vi "DMCConfiguatorGui.vi"() -> ()   [LabVIEW 2016]
uses:
  DMCConfiguatorGui.TypeGui.ctl
  DMCConfiguatorGui.VarGui.ctl
  DMCConfiguatorGui.ConfigData.ctl
  DMCConfiguatorGui.Component.ctl
  DMCConfiguatorGui.Type.ctl
  DMCConfiguatorGui.Var.ctl
  Logger/Logger.Variant.Sets.ctl
  Station/Station.Changeover.State.vi
  Station/Station.Plate.Properties.ctl
  Sequence/Sequence.Code.SerialFormat.ctl
  Drivers/V7310/LowLevel/V7310.Job.Sets.ctl
  Sequence/Sequence.PlateType.ctl
  DMCConfiguatorGui.Action.ctl
  <vilib>/Utility/miscctls.llb/LVRowAndColumnUnsignedTypeDef.ctl
  <vilib>/Utility/miscctls.llb/LVRowAndColumnTypeDef.ctl
  tools/Translator/Translator.Message.ctl
  tools/CitTemplate/citTemplate.errData.ctl
  tools/EventLog/EventLog.EventSource.ctl
  tools/Config/Config.Global.vi
  Global/ApplicationGlobal.vi
  Station/Station.Global.vi
panel:
  out "DMCconfig":i32
  out "Plate":T1
  in  "Components":i32(listbox) caption="Komponenty"
  in  "ConfigAdd":bool
  in  "ConfigInUse":i32(ring) caption="Konfiguracja" items=["Default", "975 009 005 0", "APU", "4801020307", "4801020607", "480102040R", "ceTCV", "M.KÊSKA", "cTCV", "probny", "ctcv_nrzaworu", "scania"]
  out "OrderSets":T2={"State"=enum."Init", "ImgPath"=path "", "WabcoPlate"="", "WabcoProduct"="", "ClientProduct"="", "ClientPlate"="", "TotalQuantity"=0, "OrderQuantity"=0, "Serial"=0, "Wabco"={"LaserJob"="", "AdditionalTxt"="", "FactoryCode"="037", "RevID"=0, "ForkID"=0, "FailuresLimit"=0, "GlobalCnt"=0, "ScannerProgram"=0, "SerialFormat"=enum."6 dig", "CoordA"={"X"=0.0, "Y"=0.0, "Angle"=0.0}, "CoordB"={"X"=0.0, "Y"=0.0, "Angle"=0.0}, "DMCconfig"=0, "CVX_Program"=0}, "Client"={"LaserJob"="", "AdditionalTxt"="", "FactoryCode"="037", "RevID"=0, "ForkID"=0, "FailuresLimit"=0, "GlobalCnt"=0, "ScannerProgram"=0, "SerialFormat"=enum."6 dig", "CoordA"={"X"=0.0, "Y"=0.0, "Angle"=0.0}, "CoordB"={"X"=0.0, "Y"=0.0, "Angle"=0.0}, "DMCconfig"=0, "CVX_Program"=0}}
  out "ConfigData":T7[](array[typedef])
  in  "Hider":bool
  in  "ClearAll":bool
  out "CreateDate":string
  in  "Cancel":bool
  in  "Save":bool
  in  "Down":bool
  in  "Up":bool
  in  "ConfigName":string caption="Nazwa"
  in  "ConfigDelete":bool
  out "_loop":i32(ring)=4
  in  "Delete":bool
  in  "Add":bool
  in  "Variable":T11
  in  "Text":string
  in  "Type":T12 caption="Typ"
  out "DMC":string caption="DMC (#32)"
  out "Panel":refnum<vi>
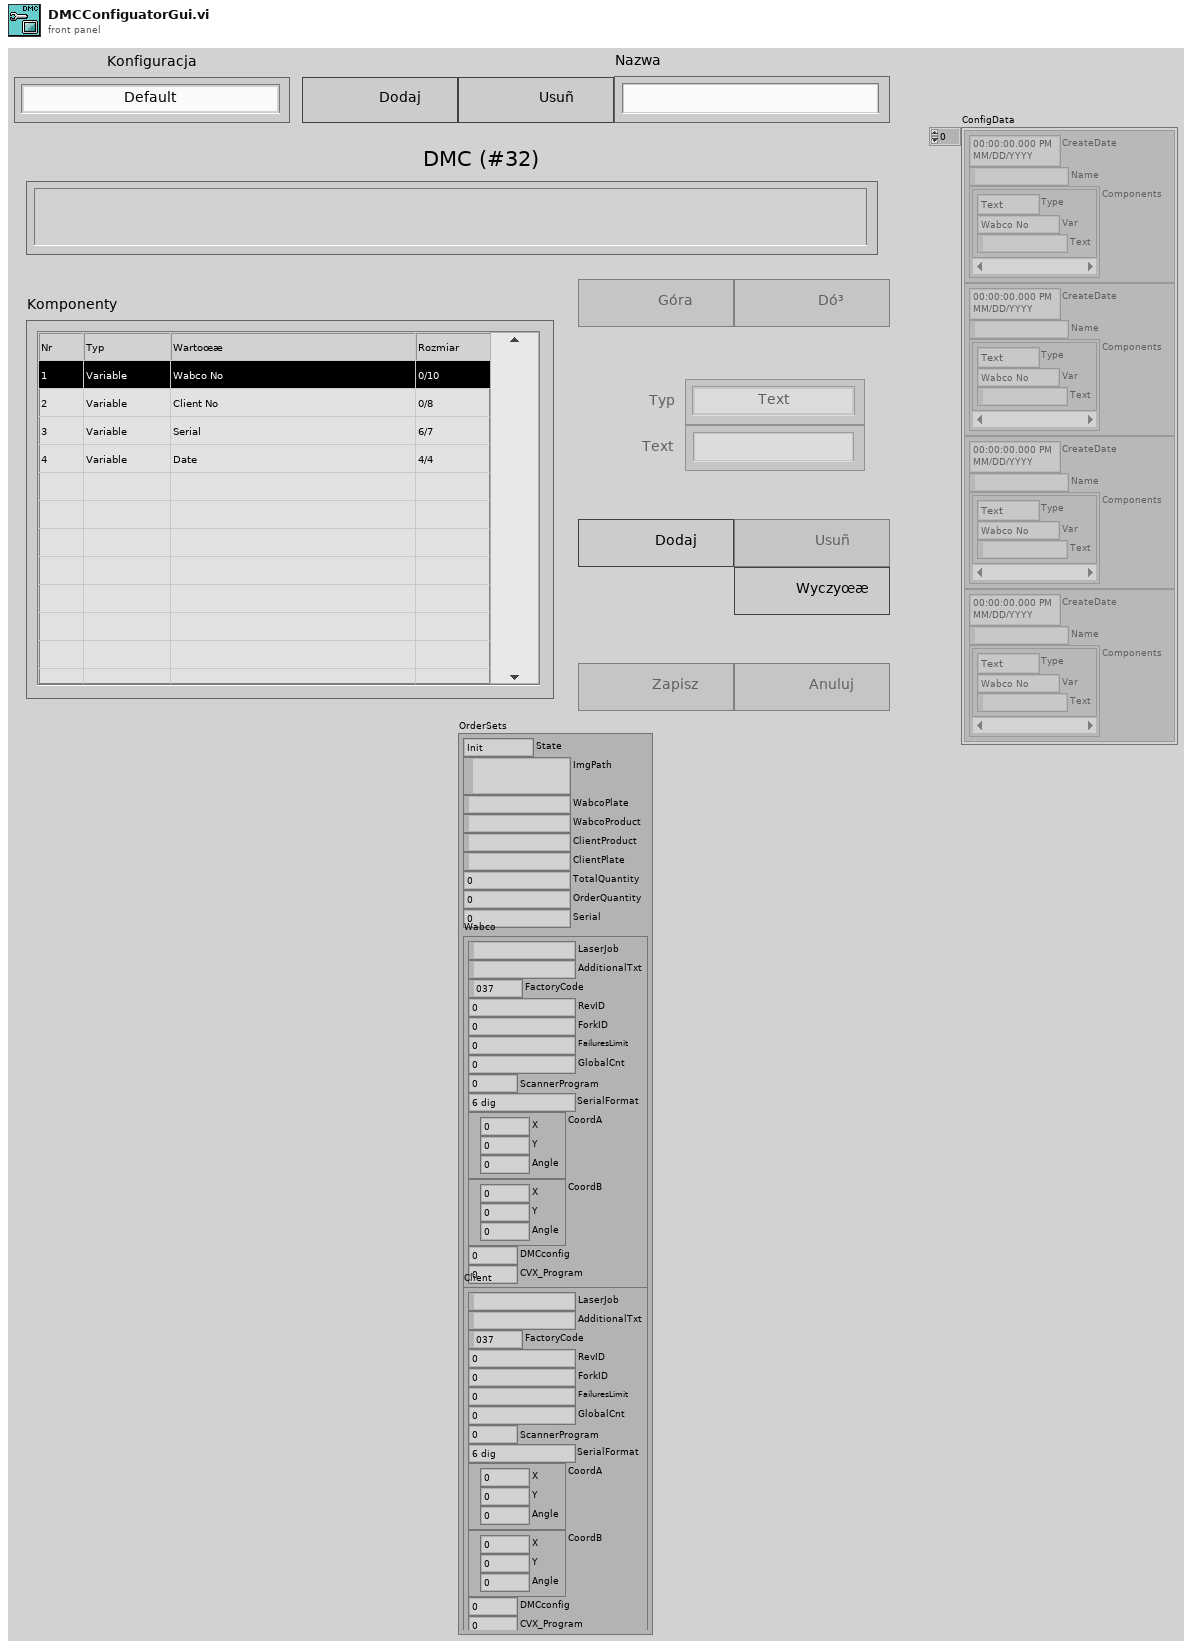
[diagram p1: front panel]
types:
  T1 = typedef "Sequence.PlateType.ctl" = enum16{"Wabco", "Client"}
  T2 = typedef "Logger.Variant.Sets.ctl" = cluster{"State":T3, "ImgPath":path, "WabcoPlate":string, "WabcoProduct":string, "ClientProduct":string, "ClientPlate":string, "TotalQuantity":u16, "OrderQuantity":u16, "Serial":i32, "Wabco":T4, "Client":T4}
  T3 = typedef "Station.Changeover.State.vi" = enum16{"Init", "Scaning", "NOK", "Wait for ack", "Ready"}
  T4 = typedef "Station.Plate.Properties.ctl" = cluster{"LaserJob":string, "AdditionalTxt":string, "FactoryCode":string, "RevID":u8, "ForkID":u8, "FailuresLimit":u16, "GlobalCnt":i32, "ScannerProgram":u8, "SerialFormat":T5, "CoordA":T6, "CoordB":T6, "DMCconfig":i32, "CVX_Program":u16}
  T5 = typedef "Sequence.Code.SerialFormat.ctl" = enum8{"", "6 dig", "7 dig"}
  T6 = typedef "V7310.Job.Sets.ctl" = cluster{"X":dbl, "Y":dbl, "Angle":dbl}
  T7 = typedef "DMCConfiguatorGui.ConfigData.ctl" = cluster{"CreateDate":timestamp, "Name":string, "Components":T8[]}
  T8 = typedef "DMCConfiguatorGui.Component.ctl" = cluster{"Type":T9, "Var":T10, "Text":string}
  T9 = typedef "DMCConfiguatorGui.Type.ctl" = enum8{"Text", "Variable"}
  T10 = typedef "DMCConfiguatorGui.Var.ctl" = enum8{"-", "Wabco No", "Client No", "Serial", "Date"}
  T11 = typedef "DMCConfiguatorGui.VarGui.ctl" = enum16{"-", "Wabco No", "Client No", "Serial", "Date"}
  T12 = typedef "DMCConfiguatorGui.TypeGui.ctl" = enum8{"Text", "Variable"}
  T13 = typedef "Translator.Message.ctl" = enum16{"-", "Event confirmed", "Log out", "Log in", "Shutdown", "Cancel", "Start", "Begin time", "End time", "Duration", "Service Mode", "Ignore Results", "Serial Format", "On", "Off", "OK", "NOK", "NOK %s", "Home", "Work", "Close", "Open", "In progress...", "Missing", "Empty", "Hardware failure", "Initial", "Default", "Total", "Out of range", "Free disk space is below 1GB - contact technician", "Error %d >> %s", "Error %d >> %s >> %s", "Msg %d >> %s", "Laser msg %d %s", "Laser cmd error %s %d", "Laser cmd failed %s", "Laser cmd warning %s", "Laser disconnected", "Laser status %s", "Laser already started", "Laser job unkonwn %s", "Laser job missing %s", "Laser job select failure %s", "Unable to start laser printing (%s)", "Unable to stop laser printing (%s)", "Laser marking aborted", "Laser marking timeout", "Unable to reset Laser Interlock (%s)", "Unable to trigger Laser. Laser not ready (%s)", "Laser job '%s' coordinates not configured", "Starting %s", "Quitting %s", "Configured", "Initializing", "Quitting", "Loading", "Loaded %d results", "Loaded %d events", "Running", "Stopped", "Summary", "Laser", "Do you want to continue?", "Do you want to delete the configuration?", "The configuration is being used by an order. Unable to delete!", "Press confirm button", "Station is not based. Do you want to exit?", "Station requires changeover. Do you want to run the test?", "Test options are not set as default. Do you want to continue?", "Formatting of WabcoNo is disabled. Do you want to continue?", "Product not detected. Do you want to continue?", "Product scan failed. Do you want to continue?", "Calibration", "Log out?", "System", "All", "IDLE", "Translating...%s", "Not found", "Alarm %s", "Run", "Skip", "Abort", "Repeat", "Please wait...", "Database disconnected", "Database disconnected - changeover disabled!", "Login to database successful", "Login to database failed: %d; %s", "Unable to check the product status of reference %d - database disconnected", "Unable to set the product status of reference %d - database disconnected", "Variant file backup %s", "Read variant (%s)", "Result", "Station armed!", "Station requires changeover!", "Select reference number...", "EMERGENCY BUTTON - press Control button", "EMERGENCY DOOR - press Control button", "Resetting Emergency...", "Unable to reset safety circuit - Emergency Button pressed", "Unable to reset safety circuit - Emergency Side Door open", "Station not based", "Station based", "Station not empty", "Station basing...", "No order", "Press Start to begin new order", "Scanning new order", "Order NOK. Correct or scan again", "Order OK. Press Accept", "Order ready", "Revolver incorrect", "Fork incorrect", "Revolver missing", "Revolver empty", "Container missing", "Offline results", "Offline statistics", "Updating statistics %.1f %%", "DMC Configurator", "Door open", "Close the front door", "Press start button", "Done. Open the front door", "Running...", "Running...%.1f %%", "Pause %s", "Pause %s. NOK container missing", "Pause %s. OK container missing", "Pause %s. Revolver empty", "Pause %s. Revolver missing", "Pause %s. Revolver incorrect", "Pause %s. Fork missing", "Pause %s. Fork incorrect", "Pause %s. Too many failures", "Pause %s. Unloading failure", "Pause %s. One slot is not working", "Pause %s. Part order is done. Empty OK container", "Pause %s. Unable to move product to slot", "Pause %s. Unable to move back product pusher", "Pause %s. Unable to lift product", "Pause %s. Unable to move back product lifter", "Pause %s. Unable to move product arm to Work", "Pause %s. Unable to move product arm to NOK", "Pause %s. Unable to move product arm to OK", "Pause %s. Unable to unsuck the NOK product", "Pause %s. Unable to drop the NOK product", "Pause %s. Product OK missing", "Pause %s. Unable to unsuck the OK product", "Pause %s. Unable to drop the OK product", "Stopping...", "File '%s' is missing", "File '%s' is broken", "File '%s' is running", "Log file started (%s)", "Log file ended (%s)", "Log file stopped (%s)", "Log file ignored (%s)", "Log file exported (%s)", "Log file export failed (%s)", "Wrong serial number in log file", "Wrong reference number in log file", "Test steps are missing", "%s = %.3f", "Process param '%s' not found in DB", "Process param '%s' wrong order", "Process param '%s' value %.3f out of limits (%.3f; %.3f)", "Step%d param '%s' not found in DB", "Step%d param '%s' wrong order", "Step%d param '%s' value %.3f out of limits (%.3f; %.3f)", "Step%d EV '%s' not found in DB", "Step%d EV '%s' wrong order", "\"%s\" not found in DB", "\"%s\" wrong order", "\"%s\" value %.3f out of limits (%.3f; %.3f)", "\"%s\" not found in software", "Process init (%s)", "Process started", "Process restarted", "Process run", "Process done", "Process done - remove OK container", "Process aborted", "Process aborted at work", "Process aborted at home", "Process error", "Process error at home", "Process error at work", "Process close", "Process pause", "Process continue", "Process door open", "Process door close", "Process pause at slot %s due to %s", "Select plate from the order to process", "Do you want to start the process?", "Do you want to continue the process?", "There is unfinished order. Do you want to put the new order?", "Product %s %d OK", "Product %s %d NOK", "Unable to unload the slot %s. Product missing in the slot", "Unable to unload the slot %s. Product already in the arm", "Unable to accept the product as OK. Product missing in slot %s", "Unable to accept the product as OK. Product could not drop into the container at slot %s", "Unable to accept the product as NOK. Product could not drop into the container at slot %s", "Scan failed. Error %s", "Scan failed. Scanner disconnected", "Scan failed. Wrong Wabco number %d, limit (%d,%d)", "Scan failed. Wrong serial number %d, limit (%d,%d)", "Scan failed. Wrong date %d, limit (%d,%d)", "Scan failed. Wrong product wabco number %d (expected %d)", "Scan failed. Wrong product serial number %d (expected > 0)", "Scan OK %s", "Scan failed. Unable to determine table position (%s)", "Scan failed. Timeout", "Tune failed. Scanner disconnected", "Tune failed. Timeout", "%s = %d", "%s = %d->%d", "Unable to set %s = %.2f - Air Pressure Inside off", "Unable to set digital output '%s' = %d", "Unable to activate air pressure inside - timeout", "Unable to activate air pressure inside - aborted", "Unable to switch on Air Main Valve - Air Pressure Inlet off", "Unable to switch on Air Main Valve - Door open", "Unable to switch off Air Main Valve - timeout", "Unable to switch off Air Main Valve - aborted", "Unable to rotate Table - timeout", "Unable to rotate Table - aborted", "Unable to rotate Table - Product Move not in Home position", "Unable to rotate Table - Air Pressure Inside off", "Unable to rotate Table - Product Lift A not in Home position", "Unable to rotate Table - Product Lift B not in Home position", "Unable to rotate Table - unlock before movement timeout", "Unable to rotate Table - lock after movement timeout", "Unable to move Table Lock to %s position - timeout", "Unable to move Table Lock to %s position - aborted", "Unable to move Table Lock to %s position - Air Pressure Inside off", "Unable to move Table Lock to %s position - Table not in position", "Unable to move Product Lift A to %s position - timeout", "Unable to move Product Lift B to %s position - timeout", "Unable to move Product Lift A to %s position - aborted", "Unable to move Product Lift B to %s position - aborted", "Unable to move Product Lift A to %s position - Air Pressure Inside off", "Unable to move Product Lift B to %s position - Air Pressure Inside off", "Unable to move Product Lift A to %s position - Table not locked", "Unable to move Product Lift B to %s position - Table not locked", "Unable to move Product Lift A to %s position - Product Arm not in Work position", "Unable to move Product Lift B to %s position - Product Arm not in Work position", "Unable to set Product Suction Gripper %s to %s - timeout", "Unable to set Product Suction Gripper %s to %s - aborted", "Unable to set Product Suction Gripper %s to %s - Air Pressure Inside off", "Unable to set Product Suction Gripper %s to %s - Table slot unkown", "Unable to move Product Arm to %s position - timeout", "Unable to move Product Arm to %s position - aborted", "Unable to move Product Arm to %s position - Air Pressure Inside off", "Unable to move Product Arm to %s position - Product Lift A not in Home position", "Unable to move Product Arm to %s position - Product Lift B not in Home position", "Unable to move Product to %s position - timeout", "Unable to move Product to %s position - aborted", "Unable to move Product to %s position - Air Pressure Inside off", "Unable to move Product to %s position - Table not in position"}
  T14 = enum8{"Enabled", "Disabled", "Disabled and Grayed Out"}
  T15 = typedef "LVRowAndColumnTypeDef.ctl" = cluster{"Row":i32, "Column":i32}
  T16 = typedef "LVRowAndColumnUnsignedTypeDef.ctl" = cluster{"Row":u32, "Column":u32}
  T17 = typedef "DMCConfiguatorGui.Action.ctl" = enum32{"idle", "constructor", "destructor", "--- DMC.Config.Gui ---", "open", "update dmc", "load configurations", "accept"}
  T18 = typedef "citTemplate.errData.ctl" = cluster{"ts":timestamp, "src":T19, "instance":i32, "action":string, "error":errorcluster, "unconfirmed":bool}
  T19 = typedef "EventLog.EventSource.ctl" = enum16{"All", "Gui", "Ref", "File", "Arch", "Seq", "CPX", "DB", "Laser", "Scan.P", "Scan.O"}
  T20 = typedef "citTemplate.notifierHandle.ctl" = refnum<notifier>
  T21 = enum32{"Invalid", "Standard", "Closed", "Hidden", "Minimized", "Maximized"}
  T22 = typedef "LVPositionTypeDef.ctl" = cluster{"Left":i32, "Top":i32}
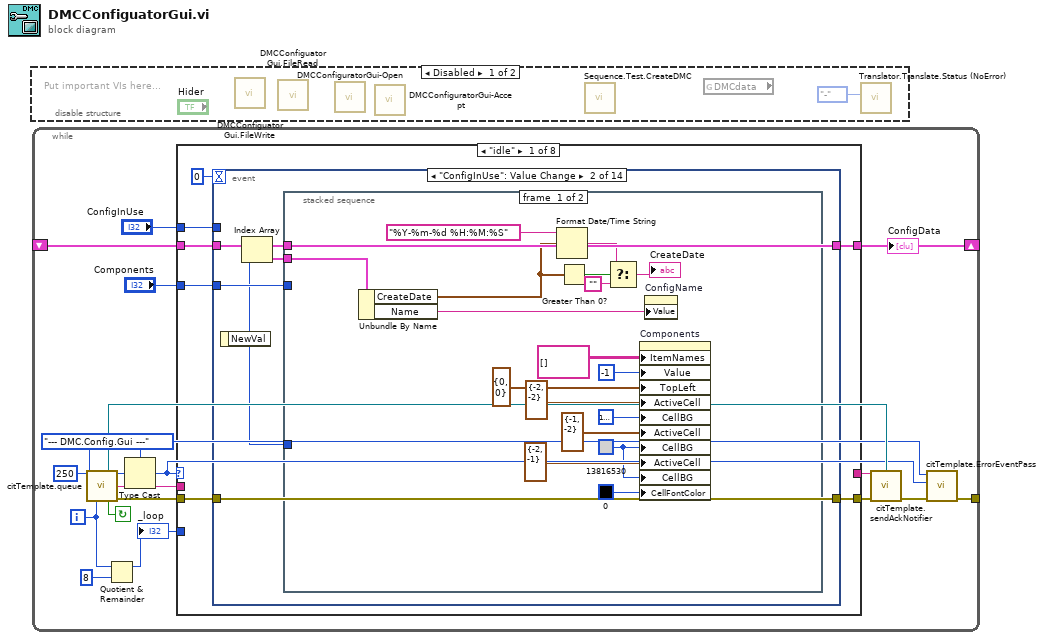
[diagram p0: block diagram]
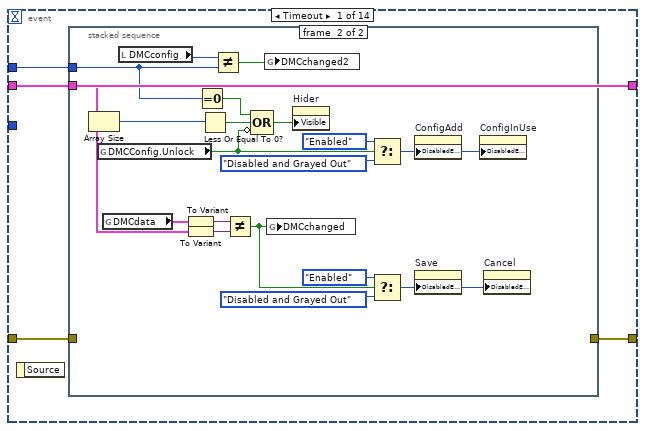
[diagram p2: hidden frame]
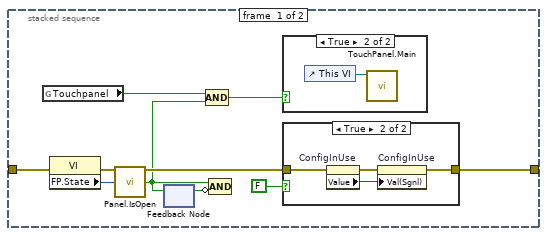
[diagram p3: hidden frame]
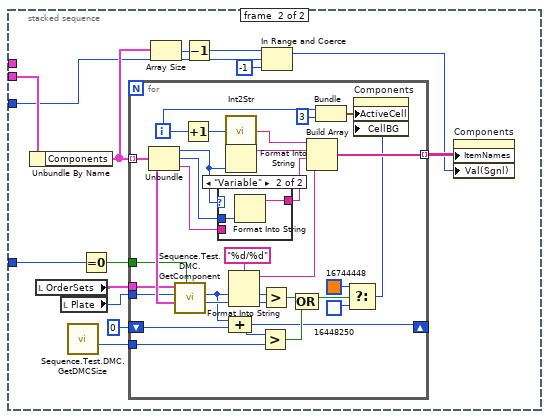
[diagram p6: hidden frame]
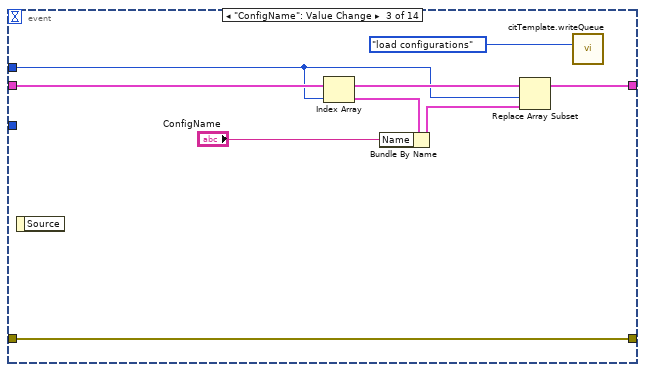
[diagram p8: hidden frame]
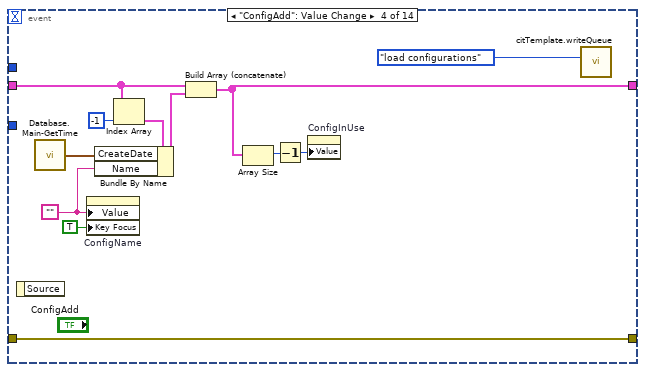
[diagram p9: hidden frame]
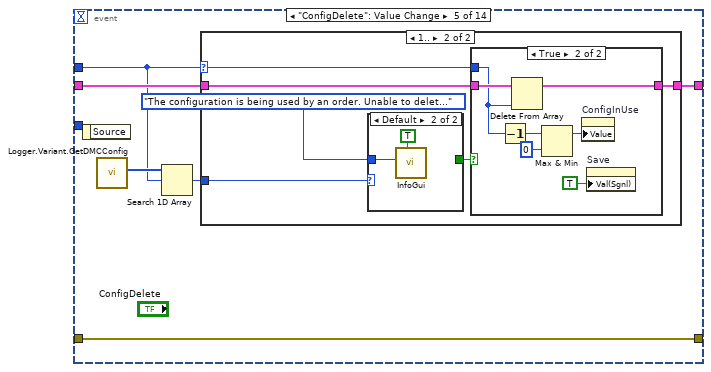
[diagram p10: hidden frame]
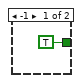
[diagram p12: hidden frame]
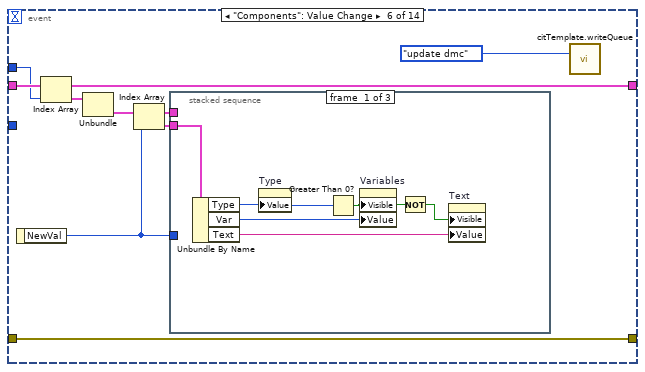
[diagram p14: hidden frame]
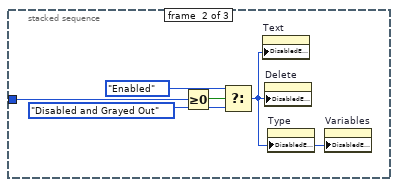
[diagram p15: hidden frame]
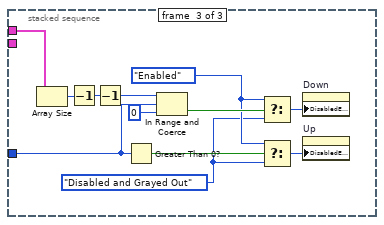
[diagram p16: hidden frame]
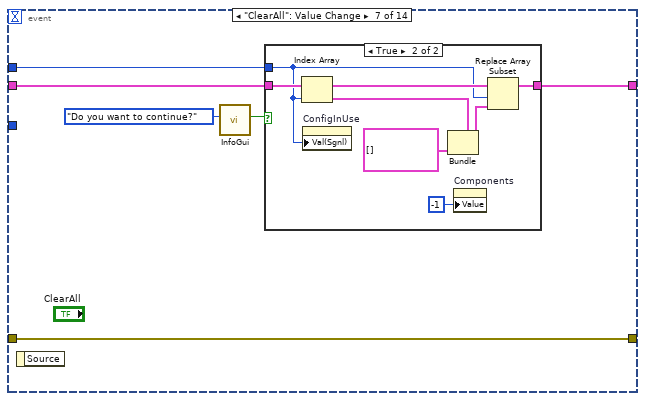
[diagram p17: hidden frame]
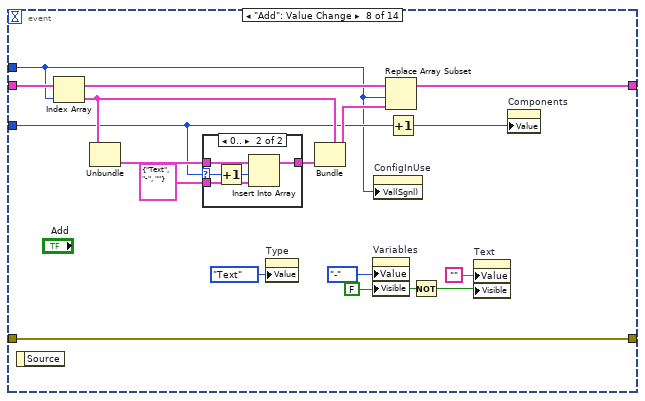
[diagram p19: hidden frame]
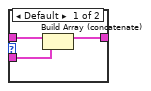
[diagram p20: hidden frame]
diagram:
  n1 = disable-structure shown="Disabled" {
    frame Disabled {
      # "Put important VIs here..."
      n2 = call "DMCConfiguatorGui.FileWrite.vi"() -> ()  [unwired: 11 in, 1 out]
      n3 = call "DMCConfiguatorGui.FileRead.vi"() -> ()  [unwired: 10 in, 2 out]
      n4 = call "DMCConfiguratorGui-Open.vi"() -> ()  [unwired: 11 in, 1 out]
      n5 = call "DMCConfiguratorGui-Accept.vi"() -> ()  [unwired: 11 in, 1 out]
      n6 = call "Sequence.Test.CreateDMC.vi"() -> ()  [unwired: 10 in, 2 out]
      n7 = global read "Station.Global.vi" "DMCdata"() -> ()  [unwired: 1 out]
      n8 = call "Translator.Translate.Status (NoError).vi"("msg"=Translator.Message."-") -> ()  [unwired: 10 in, 1 out]
    }
    frame Enabled {
    }
  }
  n9 = while {
    tunnel: [w8] -> _
    shift-right: [w5] -> _
    shift-left: _ -> [w4]
    i -> [w10]
    stop <- w16 continue-if-true
    w13 = DMCConfiguatorGui.Action."--- DMC.Config.Gui ---" ("Action")
    n10 = call "citTemplate.queue.vi"("ms timeout (250 ms)"=250, "event enum"=w13, "iteration (-1)"=w10) -> ("notifierHandle out"=w15:T20, "event out"=w19:u32, "(flatten) data out"=w18:string, "continue"=w16:bool, "error out"=w17:errorcluster)  [unwired: 2 in, 6 out]
    n11 = Quotient & Remainder(x=w10, y=8) -> (x-y*floor(x/y)=w6:i32)  [unwired: 1 out]
    "_loop" <- w6
    n12 = Type Cast(type=w13, x=w19) -> (*(type *) &x=w9:T17)
    n13 = case shown="\"idle\"" w9 {
      tunnel: w18 -> [_ _ _ w418 w431 _ _ _]
      tunnel: w17 -> [w26 w337 w391 w416 w430 w461 w484 w489]
      tunnel: [_ _ _ "" _ _ _ _] -> w14
      tunnel: [w24 w338 w392 w417 w423 w461 w484 w488] -> w12
      tunnel: w6 -> [_ _ _ _ _ _ _ _]
      tunnel: [w20 w336 w386 w412 w429 w460 w482 w490] -> w5
      tunnel: w4 -> [w23 _ w386 w412 w429 w460 w482 w490]
      tunnel: "ConfigInUse" -> [w22 _ _ _ _ w444 _ w487]
      tunnel: "Components" -> [w21 _ _ _ _ w447 _ _]
      frame "idle" {
        n14 = event shown="[1] \"ConfigInUse\": Value Change" {
          selector: _ -> [_ _ _ _ _ _ _ _ _ _ _ _ _ _]
          dyn-events: _ -> [_ _ _ _ _ _ _ _ _ _ _ _ _ _]
          timeout: 0 -> [_ _ _ _ _ _ _ _ _ _ _ _ _ _]
          tunnel: w26 -> [w30 w68 w138 w150 w155 w182 w210 w236 w250 w272 w281 w286 w287 w309]
          tunnel: [w29 w68 w138 w150 w155 w182 w210 w236 w250 w272 w280 w285 w287 w309] -> w24
          tunnel: w23 -> [w27 w66 w137 w143 w157 w183 w211 w234 w253 w268 _ w283 w294 w322]
          tunnel: w22 -> [w28 _ w136 _ w153 w181 w209 w226 w245 w256 _ _ w293 w321]
          tunnel: w21 -> [_ w67 _ _ _ _ _ w228 w246 w257 _ _ w290 w311]
          tunnel: [w27 w66 w139 w146 w156 w183 w212 w229 w254 w259 w278 w283 w291 w320] -> w20
          event Timeout {
            n15 = event-data() -> ()  [unwired: 1 in, 1 out]
            n16 = stacked-sequence {
              tunnel: w30 -> [w39 _]
              tunnel: [w35 _] -> w29
              tunnel: w28 -> [_ w48]
              tunnel: w27 -> [_ w53]
              frame #0 {
                n17 = global read "Config.Global.vi" "Touchpanel"() -> (w33:bool)
                n18 = property class="VI"(error in=w39) -> (error out=w36:errorcluster, "FP.State"=w37:T21)  [unwired: 1 in, 1 out]
                n19 = call "Panel.IsOpen.vi"("FP State"=w37) -> ("Open?"=w34:bool)
                n20 = feedback #1() -> (w38:bool)  [unwired: 1 in]
                n21 = feedback-in #1(w34) -> ()
                n22 = Compound Arithmetic op=AND(w33, w34) -> (w32:bool)
                n23 = Compound Arithmetic op=AND(w34, invert w38) -> ()  [unwired: 1 out]
                n24 = case shown="True" w32 {
                  frame False {
                  }
                  frame True {
                    n25 = control-ref of="This VI"() -> (w45:refnum<vi>)
                    n26 = call "TouchPanel.Main.vi"("VI ref"=w45) -> ()  [unwired: 8 in, 3 out]
                  }
                }
                n27 = case shown="True" FALSE {
                  tunnel: w36 -> [w40 w42]
                  tunnel: [w40 w41] -> w35
                  frame False {
                  }
                  frame True {
                    n28 = property on="ConfigInUse" class="Ring (strict)"(error in=w42) -> (error out=w43:errorcluster, "Value"=w44:i32)  [unwired: 1 in, 1 out]
                    n29 = property on="ConfigInUse" class="Ring (strict)"(error in=w43, "Val(Sgnl)"=w44) -> (error out=w41:errorcluster)  [unwired: 1 in, 1 out]
                  }
                }
              }
              frame #1 {
                n30 = Array Size(array=w53) -> (size(s)=w57:i32)
                n31 = global read "ApplicationGlobal.vi" "DMCConfig.Unlock"() -> (w61:bool)
                n32 = global read "Station.Global.vi" "DMCdata"() -> (w56:T7[])
                n33 = local read "DMCconfig"() -> (w47:i32)
                n34 = To Variant(anything=w56) -> (Variant=w55:variant)
                n35 = To Variant(anything=w53) -> (Variant=w54:variant)
                n36 = Equal To 0?(x=w48) -> (x = 0?=w60:bool)
                n37 = Less Or Equal To 0?(x=w57) -> (x <= 0?=w58:bool)
                n38 = Not Equal?(x=w47, y=w48) -> (x != y?=w46:bool)
                n39 = Not Equal?(x=w55, y=w54) -> (x != y?=w51:bool)
                n40 = Compound Arithmetic op=OR(w60, w58, invert w61) -> (w59:bool)
                n41 = global write "Station.Global.vi" "DMCchanged2"(w46) -> ()
                n42 = global write "Station.Global.vi" "DMCchanged"(w51) -> ()
                n43 = property on="Hider" class="Bool (strict)"("Visible"=w59) -> ()  [unwired: 2 in, 2 out]
                n44 = Select(t=T14."Enabled" ("Disabled"), s=w61, f=T14."Disabled and Grayed Out" ("Disabled")) -> (s? t:f=w64:T14)
                n45 = Select(t=T14."Enabled" ("Disabled"), s=w51, f=T14."Disabled and Grayed Out" ("Disabled")) -> (s? t:f=w49:T14)
                n46 = property on="ConfigAdd" class="Bool"("DisabledEnum"=w64) -> ()  [unwired: 2 in, 2 out]
                n47 = property on="Save" class="Bool (strict)"("DisabledEnum"=w49) -> ()  [unwired: 2 in, 2 out]
                n48 = property on="ConfigInUse" class="Ring (strict)"("DisabledEnum"=w64) -> ()  [unwired: 2 in, 2 out]
                n49 = property on="Cancel" class="Bool (strict)"("DisabledEnum"=w49) -> ()  [unwired: 2 in, 2 out]
              }
            }
          }
          event "ConfigInUse": Value Change {
            n50 = event-data() -> ("NewVal"=w65:i32)  [unwired: 1 in]
            n51 = Index Array(array=w66, index=w65) -> (element=w69:T7)
            n52 = stacked-sequence {
              tunnel: w69 -> [w85 w100]
              tunnel: w67 -> [_ w91]
              tunnel: w66 -> [_ _]
              tunnel: w65 -> [_ w87]
              frame #0 {
                w70 = u32 13816530
                n53 = Unbundle By Name(w85) -> ("CreateDate"=w79:timestamp, "Name"=w84:string)
                n54 = Format Date/Time String(time format string (%c)="%Y-%m-%d %H:%M:%S", seconds (now)=w79) -> (date/time string=w83:string)  [unwired: 1 in]
                n55 = Greater Than 0?(x=w79) -> (x > 0?=w80:bool)
                n56 = Select(t=w83, s=w80, f="") -> (s? t:f=→"CreateDate":string)
                n57 = property on="Components" class="MCListbox (strict)"("ItemNames"=string[][] [] ("Item Names"), "Value"=-1 ("Properties"), "TopLeft"=T16 {"Row"=0, "Column"=0} ("Top Left Visible Cell"), "ActiveCell"=T15 {"Row"=-2, "Column"=-2} ("Active Cell:Active Cell"), "CellBG"=u32 16777225, "ActiveCell"=T15 {"Row"=-1, "Column"=-2} ("Active Cell:Active Cell"), "CellBG"=w70, "ActiveCell"=T15 {"Row"=-2, "Column"=-1} ("Active Cell:Active Cell"), "CellBG"=w70, "CellFontColor"=u32 0) -> ()  [unwired: 2 in, 2 out]
                n58 = property on="ConfigName" class="Str"("Value"=w84) -> ()  [unwired: 2 in, 2 out]
              }
              frame #1 {
                n59 = Unbundle By Name(w100) -> ("Components"=w95:T8[])
                n60 = local read "OrderSets"() -> (w93:T2)
                n61 = local read "Plate"() -> (w92:T1)
                n62 = call "Sequence.Test.DMC.GetDMCSize.vi"() -> ("max size"=w88:i32)  [unwired: 11 in]
                n63 = Equal To 0?(x=w87) -> (x = 0?=w90:bool)
                n64 = for {
                  tunnel: w95 -> [w120] mode=indexing
                  tunnel: [w128] -> w99 mode=indexing
                  tunnel: w92 -> [w119]
                  tunnel: w93 -> [w118]
                  tunnel: w90 -> [w107]
                  shift-right: [w101] -> _
                  shift-left: 0 -> [w105]
                  tunnel: w88 -> [w104]
                  i -> [w111]
                  n65 = Unbundle(w120) -> ("Type"=w121:T9, "Var"=w123:T10, "Text"=w124:string)
                  n66 = call "Sequence.Test.DMC.GetComponent.vi"("Default"=w107, "Component"=w120, "Plate"=w119, "OrderSets"=w118) -> ("max size"=w115:i32, "size"=w106:i32)  [unwired: 5 in, 1 out]
                  n67 = Increment(x=w111) -> (x+1=w125:i32)
                  n68 = case shown="\"Variable\"" w121 {
                    tunnel: w123 -> [_ w130]
                    tunnel: w124 -> [w129 _]
                    tunnel: [w129 w131] -> w122
                    frame "Text" {
                    }
                    frame "Variable" {
                      n69 = Format Into String(w130) -> (resulting string=w131:string)  [unwired: 3 in, 1 out]
                    }
                  }
                  n70 = call "Int2Str.vi"("Numeric"=w125) -> ("string"=w126:string)
                  n71 = Format Into String(w121) -> (resulting string=w127:string)  [unwired: 3 in, 1 out]
                  n72 = Format Into String(format string="%d/%d", w106, w115) -> (resulting string=w116:string)  [unwired: 2 in, 1 out]
                  n73 = Compound Arithmetic op=ADD(w106, w105) -> (w101:i32)
                  n74 = Greater?(x=w101, y=w104) -> (0:w102:bool)
                  n75 = Greater?(x=w106, y=w115) -> (0:w114:bool)
                  n76 = Compound Arithmetic op=OR(w114, w102) -> (w103:bool)
                  n77 = Build Array(w126, w127, w122, w116) -> (w128:string[])
                  n78 = Bundle(w111, 3) -> (w109:cluster{i32, i32})  [unwired: 1 in]
                  n79 = Select(t=u32 16744448, s=w103, f=u32 16448250) -> (s? t:f=w108:u32)
                  n80 = property on="Components" class="MCListbox (strict)"("ActiveCell"=w109, "CellBG"=w108) -> ()  [unwired: 2 in, 2 out]
                }
                n81 = Array Size(array=w95) -> (size(s)=w98:i32)
                n82 = Decrement(x=w98) -> (x-1=w96:i32)
                n83 = In Range and Coerce(upper limit=w96, x=w91, lower limit=-1) -> (coerced(x)=w94:i32)  [unwired: 1 out]
                n84 = property on="Components" class="MCListbox (strict)"("ItemNames"=w99, "Val(Sgnl)"=w94) -> ()  [unwired: 2 in, 2 out]
              }
            }
          }
          event "ConfigName": Value Change {
            n85 = event-data() -> ()  [unwired: 1 in, 1 out]
            n86 = Index Array(array=w137, index=w136) -> (element=w135:T7)
            n87 = Bundle By Name(cluster=w135, "Name"="ConfigName") -> (w134:T7)
            n88 = Replace Array Subset(array=w137, new element=w134, index=w136) -> (w139:T7[])
            n89 = call "citTemplate.writeQueue.vi"("event in (if not connected:all statemachine with data event)"=DMCConfiguatorGui.Action."load configurations" ("Action")) -> ()  [unwired: 14 in, 1 out]
          }
          event "ConfigAdd": Value Change {
            w142 = ""
            n90 = event-data() -> ()  [unwired: 1 in, 1 out]
            n91 = call "Database.Main-GetTime.vi"() -> ("TS"=w140:timestamp)  [unwired: 1 in]
            n92 = property on="ConfigName" class="Str"("Value"=w142, "Key Focus"=TRUE) -> ()  [unwired: 2 in, 2 out]
            n93 = Index Array(array=w143, index=-1) -> (element=w145:T7)
            n94 = Bundle By Name(cluster=w145, "CreateDate"=w140, "Name"=w142) -> (w144:T7)
            n95 = Build Array (concatenate)(w143, w144) -> (w146:T7[])
            n96 = Array Size(array=w146) -> (size(s)=w149:i32)
            n97 = Decrement(x=w149) -> (x-1=w148:i32)
            n98 = property on="ConfigInUse" class="Ring (strict)"("Value"=w148) -> ()  [unwired: 2 in, 2 out]
            n99 = call "citTemplate.writeQueue.vi"("event in (if not connected:all statemachine with data event)"=DMCConfiguatorGui.Action."load configurations" ("Action")) -> ()  [unwired: 14 in, 1 out]
          }
          event "ConfigDelete": Value Change {
            n100 = event-data() -> ()  [unwired: 1 in, 1 out]
            n101 = call "Logger.Variant.GetDMCConfig.vi"() -> ("DMCconfig"=w154:i32[])  [unwired: 10 in, 1 out]
            n102 = Search 1D Array(1D array=w154, element=w153) -> (index of element=w152:i32)  [unwired: 1 in]
            n103 = case shown="1.." w153 {
              selector: w153 -> [_ w162]
              tunnel: w157 -> [w158 w164]
              tunnel: [w158 w163] -> w156
              tunnel: w152 -> [_ w159]
              frame Default {
              }
              frame 1.. {
                n104 = case shown="Default" w159 {
                  tunnel: [TRUE ("ok") _] -> w161
                  tunnel: Translator.Message."The configuration is being used by an order. Unable to delete!" ("msg") -> [_ w167]
                  frame -1 {
                  }
                  frame Default {
                    n105 = call "InfoGui.vi"("_onebutton(F)"=TRUE, "_Msg"=w167) -> ()  [unwired: 9 in, 1 out]
                  }
                }
                n106 = case shown="True" w161 {
                  tunnel: w164 -> [w168 w175]
                  tunnel: [w168 w174] -> w163
                  tunnel: w162 -> [_ w170]
                  frame False {
                  }
                  frame True {
                    n107 = Decrement(x=w170) -> (x-1=w173:i32)
                    n108 = Delete From Array(array=w175, index=w170) -> (array with subset deleted=w174:T7[])  [unwired: 1 in, 1 out]
                    n109 = Max & Min(x=w173, y=0) -> (max(x,y)=w172:i32)  [unwired: 1 out]
                    n110 = property on="ConfigInUse" class="Ring (strict)"("Value"=w172) -> ()  [unwired: 2 in, 2 out]
                    n111 = property on="Save" class="Bool (strict)"("Val(Sgnl)"=TRUE ("Value (Signaling)")) -> ()  [unwired: 2 in, 2 out]
                  }
                }
              }
            }
          }
          event "Components": Value Change {
            n112 = event-data() -> ("NewVal"=w177:i32)  [unwired: 1 in]
            n113 = Index Array(array=w183, index=w181) -> (element=w180:T7)
            n114 = Unbundle(w180) -> ("Components"=w178:T8[])  [unwired: 2 out]
            n115 = Index Array(array=w178, index=w177) -> (element=w179:T8)
            n116 = stacked-sequence {
              tunnel: w179 -> [w184 _ _]
              tunnel: w177 -> [_ w193 w201]
              tunnel: w178 -> [_ _ w202]
              frame #0 {
                n117 = Unbundle By Name(w184) -> ("Type"=w187:T9, "Var"=w189:T10, "Text"=w185:string)
                n118 = property on="Type" class="Enum (strict)"("Value"=w187) -> ()  [unwired: 2 in, 2 out]
                n119 = Greater Than 0?(x=w187) -> (x > 0?=w186:bool)
                n120 = property on="Variables" class="Enum (strict)"("Visible"=w186, "Value"=w189) -> ()  [unwired: 2 in, 2 out]
                n121 = Not(x=w186) -> (.not. x?=w188:bool)
                n122 = property on="Text" class="Str"("Visible"=w188, "Value"=w185) -> ()  [unwired: 2 in, 2 out]
              }
              frame #1 {
                n123 = Greater Or Equal To 0?(x=w193) -> (x >= 0?=w194:bool)
                n124 = Select(t=T14."Enabled" ("Disabled"), s=w194, f=T14."Disabled and Grayed Out" ("Disabled")) -> (s? t:f=w190:T14)
                n125 = property on="Text" class="Str"("DisabledEnum"=w190) -> ()  [unwired: 2 in, 2 out]
                n126 = property on="Delete" class="Bool"("DisabledEnum"=w190) -> ()  [unwired: 2 in, 2 out]
                n127 = property on="Type" class="Enum (strict)"("DisabledEnum"=w190) -> ()  [unwired: 2 in, 2 out]
                n128 = property on="Variables" class="Enum (strict)"("DisabledEnum"=w190) -> ()  [unwired: 2 in, 2 out]
              }
              frame #2 {
                w195 = T14."Disabled and Grayed Out" ("Disabled")
                w197 = T14."Enabled" ("Disabled")
                n129 = Array Size(array=w202) -> (size(s)=w205:i32)
                n130 = Decrement(x=w205) -> (x-1=w204:i32)
                n131 = Decrement(x=w204) -> (x-1=w203:i32)
                n132 = Greater Than 0?(x=w201) -> (x > 0?=w196:bool)
                n133 = In Range and Coerce(upper limit=w203, x=w201, lower limit=0) -> (In Range?=w200:bool)  [unwired: 1 out]
                n134 = Select(t=w197, s=w200, f=w195) -> (s? t:f=w199:T14)
                n135 = Select(t=w197, s=w196, f=w195) -> (s? t:f=w198:T14)
                n136 = property on="Down" class="Bool"("DisabledEnum"=w199) -> ()  [unwired: 2 in, 2 out]
                n137 = property on="Up" class="Bool"("DisabledEnum"=w198) -> ()  [unwired: 2 in, 2 out]
              }
            }
            n138 = call "citTemplate.writeQueue.vi"("event in (if not connected:all statemachine with data event)"=DMCConfiguatorGui.Action."update dmc" ("Action")) -> ()  [unwired: 14 in, 1 out]
          }
          event "ClearAll": Value Change {
            n139 = event-data() -> ()  [unwired: 1 in, 1 out]
            n140 = call "InfoGui.vi"("_Msg"=Translator.Message."Do you want to continue?" ("msg")) -> ("ok"=w207:bool)  [unwired: 10 in]
            n141 = case shown="True" w207 {
              tunnel: [w213 w219] -> w212
              tunnel: w211 -> [w213 w218]
              tunnel: w209 -> [_ w215]
              frame False {
              }
              frame True {
                n142 = Index Array(array=w218, index=w215) -> (element=w217:T7)
                n143 = property on="ConfigInUse" class="Ring (strict)"("Val(Sgnl)"=w215) -> ()  [unwired: 2 in, 2 out]
                n144 = Bundle(cluster=w217, "Components"=T8[] []) -> (w220:T7)  [unwired: 2 in]
                n145 = property on="Components" class="MCListbox (strict)"("Value"=-1 ("Components")) -> ()  [unwired: 2 in, 2 out]
                n146 = Replace Array Subset(array=w218, new element=w220, index=w215) -> (w219:T7[])
              }
            }
          }
          event "Add": Value Change {
            w222 = FALSE ("Visible")
            n147 = event-data() -> ()  [unwired: 1 in, 1 out]
            n148 = Index Array(array=w234, index=w226) -> (element=w233:T7)
            n149 = Unbundle(w233) -> ("Components"=w232:T8[])  [unwired: 2 out]
            n150 = case shown="0.." w228 {
              selector: w228 -> [_ w241]
              tunnel: w232 -> [w239 w244]
              tunnel: [w237 w243] -> w231
              tunnel: T8 {"Type"=enum."Text", "Var"=enum."-", "Text"=""} ("new element/subarray") -> [w238 w242]
              frame Default {
                n151 = Build Array (concatenate)(w239, w238) -> (w237:T8[])
              }
              frame 0.. {
                n152 = Increment(x=w241) -> (x+1=w240:i32)
                n153 = Insert Into Array(array=w244, index=w240, new element=w242) -> (w243:T8[])
              }
            }
            n154 = property on="Type" class="Enum (strict)"("Value"=DMCConfiguatorGui.TypeGui."Text" ("Type")) -> ()  [unwired: 2 in, 2 out]
            n155 = Bundle(cluster=w233, "Components"=w231) -> (w235:T7)  [unwired: 2 in]
            n156 = property on="Variables" class="Enum (strict)"("Value"=DMCConfiguatorGui.VarGui."-" ("Variable"), "Visible"=w222) -> ()  [unwired: 2 in, 2 out]
            n157 = property on="ConfigInUse" class="Ring (strict)"("Val(Sgnl)"=w226) -> ()  [unwired: 2 in, 2 out]
            n158 = Replace Array Subset(array=w234, new element=w235, index=w226) -> (w229:T7[])
            n159 = Increment(x=w228) -> (x+1=w230:i32)
            n160 = Not(x=w222) -> (.not. x?=w221:bool)
            n161 = property on="Text" class="Str"("Value"="", "Visible"=w221) -> ()  [unwired: 2 in, 2 out]
            n162 = property on="Components" class="MCListbox (strict)"("Value"=w230) -> ()  [unwired: 2 in, 2 out]
          }
          event "Delete": Value Change {
            n163 = event-data() -> ()  [unwired: 1 in, 1 out]
            n164 = Index Array(array=w253, index=w245) -> (element=w251:T7)
            n165 = Unbundle(w251) -> ("Components"=w249:T8[])  [unwired: 2 out]
            n166 = Delete From Array(array=w249, index=w246) -> (array with subset deleted=w248:T8[])  [unwired: 1 in, 1 out]
            n167 = Decrement(x=w246) -> (x-1=w247:i32)
            n168 = Bundle(cluster=w251, "Components"=w248) -> (w252:T7)  [unwired: 2 in]
            n169 = property on="Components" class="MCListbox (strict)"("Value"=w247) -> ()  [unwired: 2 in, 2 out]
            n170 = Replace Array Subset(array=w253, new element=w252, index=w245) -> (w254:T7[])
            n171 = property on="ConfigInUse" class="Ring (strict)"("Val(Sgnl)"=w245) -> ()  [unwired: 2 in, 2 out]
          }
          event "Text": Value Change {
            n172 = event-data() -> ()  [unwired: 1 in, 1 out]
            n173 = Index Array(array=w268, index=w256) -> (element=w270:T7)
            n174 = Unbundle(w270) -> ("Components"=w267:T8[])  [unwired: 2 out]
            n175 = Index Array(array=w267, index=w257) -> (element=w266:T8)
            n176 = Search and Replace String(replace all?=TRUE ("replace all? (F)"), input string="Text", search string=";" ("replace string (\"\")")) -> (result string=w260:string)  [unwired: 5 in, 3 out]
            n177 = call <vilib>:"Trim Whitespace.vi"("string"=w260) -> ("trimmed string"=w255:string)  [unwired: 1 in]
            n178 = Bundle(cluster=w266, "Type"="Type", "Var"="Variable", "Text"=w255) -> (w265:T8)
            n179 = case shown="\"Text\"" "Type" {
              tunnel: [_ TRUE] -> w274
              tunnel: [TRUE _] -> w273
              frame "Text" {
              }
              frame "Variable" {
              }
            }
            n180 = Replace Array Subset(array=w267, new element=w265, index=w257) -> (w269:T8[])
            n181 = Bundle(cluster=w270, "Components"=w269) -> (w271:T7)  [unwired: 2 in]
            n182 = property on="Variables" class="Enum (strict)"("Visible"=w274) -> ()  [unwired: 2 in, 2 out]
            n183 = property on="Text" class="Str"("Visible"=w273) -> ()  [unwired: 2 in, 2 out]
            n184 = Replace Array Subset(array=w268, new element=w271, index=w256) -> (w259:T7[])
            n185 = property on="ConfigInUse" class="Ring (strict)"("Val(Sgnl)"=w256) -> ()  [unwired: 2 in, 2 out]
          }
          event "Cancel": Value Change {
            n186 = event-data() -> ()  [unwired: 1 in, 1 out]
            n187 = call "DMCConfiguatorGui.FileRead.vi"("error in (no error)"=w281) -> ("error out"=w280:errorcluster, "ConfigData"=w278:T7[])  [unwired: 9 in]
            n188 = global write "Station.Global.vi" "DMCdata"(w278) -> ()
            n189 = property on="Cancel" class="Bool (strict)"("Value"=FALSE ("Cancel")) -> ()  [unwired: 2 in, 2 out]
            n190 = call "citTemplate.writeQueue.vi"("event in (if not connected:all statemachine with data event)"=DMCConfiguatorGui.Action."load configurations" ("Action")) -> ()  [unwired: 14 in, 1 out]
          }
          event "Save": Value Change {
            n191 = event-data() -> ()  [unwired: 1 in, 1 out]
            n192 = global write "Station.Global.vi" "DMCdata"(w283) -> ()
            n193 = call "DMCConfiguatorGui.FileWrite.vi"("error in (no error)"=w286, "ConfigData"=w283) -> ("error out"=w285:errorcluster)  [unwired: 9 in]
            n194 = property on="Save" class="Bool (strict)"("Value"=FALSE ("Value (Signaling)")) -> ()  [unwired: 2 in, 2 out]
            n195 = call "citTemplate.writeQueue.vi"("event in (if not connected:all statemachine with data event)"=DMCConfiguatorGui.Action."load configurations" ("Action")) -> ()  [unwired: 14 in, 1 out]
          }
          event "Up": Value Change {
            n196 = event-data() -> ()  [unwired: 1 in, 1 out]
            n197 = Index Array(array=w294, index=w293) -> (element=w296:T7)
            n198 = Unbundle(w296) -> ("Components"=w295:T8[])  [unwired: 2 out]
            n199 = Decrement(x=w290) -> (x-1=w292:i32)
            n200 = Index Array(array=w295, index #1=w292, index #2=w290) -> (element #1=w289:T8, element #2=w288:T8)
            n201 = case shown="1.." w290 {
              selector: w290 -> [_ w302]
              tunnel: w296 -> [_ w307]
              tunnel: w295 -> [_ w305]
              tunnel: w294 -> [w297 w304]
              tunnel: w293 -> [_ w298]
              tunnel: [w297 w303] -> w291
              tunnel: w289 -> [_ w301]
              tunnel: w288 -> [_ w300]
              frame Default {
              }
              frame 1.. {
                n202 = Decrement(x=w302) -> (x-1=w299:i32)
                n203 = Replace Array Subset(array=w305, new element #1=w301, index #1=w302, new element #2=w300, index #2=w299) -> (w306:T8[])
                n204 = Bundle(cluster=w307, "Components"=w306) -> (w308:T7)  [unwired: 2 in]
                n205 = Replace Array Subset(array=w304, new element=w308, index=w298) -> (w303:T7[])
                n206 = property on="Components" class="MCListbox (strict)"("Value"=w299) -> ()  [unwired: 2 in, 2 out]
                n207 = property on="ConfigInUse" class="Ring (strict)"("Val(Sgnl)"=w298) -> ()  [unwired: 2 in, 2 out]
              }
            }
          }
          event "Down": Value Change {
            n208 = event-data() -> ()  [unwired: 1 in, 1 out]
            n209 = Index Array(array=w322, index=w321) -> (element=w323:T7)
            n210 = Unbundle(w323) -> ("Components"=w316:T8[])  [unwired: 2 out]
            n211 = Array Size(array=w316) -> (size(s)=w315:i32)
            n212 = Decrement(x=w315) -> (x-1=w314:i32)
            n213 = Decrement(x=w314) -> (x-1=w313:i32)
            n214 = Increment(x=w311) -> (x+1=w312:i32)
            n215 = In Range and Coerce(upper limit=w313, x=w311, lower limit=0) -> (In Range?=w310:bool)  [unwired: 1 out]
            n216 = Index Array(array=w316, index #1=w311, index #2=w312) -> (element #1=w319:T8, element #2=w318:T8)
            n217 = case shown="True" w310 {
              tunnel: w323 -> [_ w334]
              tunnel: w316 -> [_ w332]
              tunnel: w322 -> [w324 w331]
              tunnel: w321 -> [_ w325]
              tunnel: [w324 w330] -> w320
              tunnel: w319 -> [_ w329]
              tunnel: w318 -> [_ w328]
              tunnel: w311 -> [_ w327]
              frame False {
              }
              frame True {
                n218 = Increment(x=w327) -> (x+1=w326:i32)
                n219 = Replace Array Subset(array=w332, new element #1=w329, index #1=w326, new element #2=w328, index #2=w327) -> (w333:T8[])
                n220 = Bundle(cluster=w334, "Components"=w333) -> (w335:T7)  [unwired: 2 in]
                n221 = Replace Array Subset(array=w331, new element=w335, index=w325) -> (w330:T7[])
                n222 = property on="Components" class="MCListbox (strict)"("Value"=w326) -> ()  [unwired: 2 in, 2 out]
                n223 = property on="ConfigInUse" class="Ring (strict)"("Val(Sgnl)"=w325) -> ()  [unwired: 2 in, 2 out]
              }
            }
          }
        }
      }
      frame "constructor" {
        n224 = stacked-sequence {
          tunnel: [_ _ w376 _] -> w338
          tunnel: w337 -> [_ _ w377 _]
          tunnel: [_ _ _ T7[] [] ("ConfigData")] -> w336
          frame #0 {
            n225 = control-ref of="This VI"() -> (w344:refnum<vi>)
            n226 = property class="VI"(reference=w344) -> (reference out=w343:refnum<vi>, error out=w342:errorcluster, "Front Panel"=→"Panel":refnum<vi>, "FP.State"=w341:T21)  [unwired: 1 in]
            n227 = property on="_loop" class="Ring (strict)"() -> (error out=w346:errorcluster, "Position"=w345:T22)  [unwired: 2 in, 1 out]
            n228 = case shown="\"Standard\", \"Minimized\", \"Maximized\"" w341 {
              tunnel: w343 -> [w348 w352]
              tunnel: w342 -> [w347 w351]
              tunnel: [w348 w350] -> w340
              tunnel: [w347 w349] -> _
              frame Default {
              }
              frame "Standard", "Minimized", "Maximized" {
                n229 = disable-structure shown="Disabled" {
                  disable-tunnel: w352 -> [w356 w357]
                  disable-tunnel: w351 -> [w355 w358]
                  disable-tunnel: [w354 w357] -> w350
                  disable-tunnel: [w353 w358] -> w349
                  frame Enabled {
                    n230 = invoke class="VI" method="FP.Close"(reference=w356, error in=w355) -> (reference out=w354:refnum<vi>, error out=w353:errorcluster)  [unwired: 1 in, 1 out]
                  }
                  frame Disabled {
                  }
                }
              }
            }
            n231 = property on="Pane" class="Pane"(error in=w346, "Origin"=w345) -> ()  [unwired: 1 in, 2 out]
            n232 = global write "ApplicationGlobal.vi" "GuiRef.DMCConfig"(w340) -> ()
          }
          frame #1 {
            w359 = T14."Disabled and Grayed Out" ("Disabled")
            w361 = TRUE ("Visible")
            w367 = u32 13816530
            n233 = property on="Components" class="MCListbox (strict)"("ItemNames"=string[][] [] ("Item Names"), "Value"=-1 ("Properties"), "TopLeft"=T16 {"Row"=0, "Column"=0} ("Top Left Visible Cell"), "ActiveCell"=T15 {"Row"=-2, "Column"=-2} ("Active Cell:Active Cell"), "CellBG"=u32 16777225, "ActiveCell"=T15 {"Row"=-1, "Column"=-2} ("Active Cell:Active Cell"), "CellBG"=w367, "ActiveCell"=T15 {"Row"=-2, "Column"=-1} ("Active Cell:Active Cell"), "CellBG"=w367, "CellFontColor"=u32 0) -> ()  [unwired: 2 in, 2 out]
            n234 = property on="Type" class="Enum (strict)"("Value"=DMCConfiguatorGui.TypeGui."Text" ("Type")) -> (error out=w364:errorcluster)  [unwired: 2 in, 1 out]
            n235 = property on="Text" class="Str"(error in=w364, "Value"="", "Visible"=w361) -> (error out=w363:errorcluster)  [unwired: 1 in, 1 out]
            n236 = property on="Variables" class="Enum (strict)"(error in=w363, "Value"=DMCConfiguatorGui.VarGui."-" ("Variables"), "Visible"=w361) -> ()  [unwired: 1 in, 2 out]
            n237 = property on="ConfigAdd" class="Bool"("DisabledEnum"=w359) -> ()  [unwired: 2 in, 2 out]
            n238 = property on="ConfigInUse" class="Ring (strict)"("DisabledEnum"=w359) -> ()  [unwired: 2 in, 2 out]
            n239 = property on="Hider" class="Bool (strict)"("Visible"=TRUE) -> ()  [unwired: 2 in, 2 out]
          }
          frame #2 {
            n240 = call "Translator.TranslateThis.Init.vi"("error in"=w377) -> ("error out"=w376:errorcluster)  [unwired: 10 in]
          }
          frame #3 {
            n241 = property on="Type" class="Enum (strict)"() -> ("Value"=w382:T12)  [unwired: 2 in, 2 out]
            n242 = Equal?(x=w382, y=DMCConfiguatorGui.TypeGui."Text") -> (x = y?=w380:bool)
            n243 = disable-structure shown="Disabled" {
              frame Disabled {
                n244 = while {
                  stop <- w385 stop-if-true
                  n245 = global read "ApplicationGlobal.vi" "AppLaunched"() -> (w385:bool)
                  n246 = Wait (ms)(milliseconds to wait=u32 50) -> ()  [unwired: 1 out]
                }
              }
              frame Enabled {
              }
            }
            n247 = property on="Text" class="Str"("Visible"=w380) -> ()  [unwired: 2 in, 2 out]
            n248 = property on="Cancel" class="Bool (strict)"("Val(Sgnl)"=FALSE ("Value (Signaling)")) -> ()  [unwired: 2 in, 2 out]
            n249 = Not(x=w380) -> (.not. x?=w383:bool)
            n250 = property on="Variables" class="Enum (strict)"("Visible"=w383) -> ()  [unwired: 2 in, 2 out]
          }
        }
      }
      frame "destructor" {
        n251 = local read "Panel"() -> (w387:refnum<vi>)
        n252 = stacked-sequence {
          tunnel: [_ w411] -> w392
          tunnel: w391 -> [_ w410]
          frame #0 {
            w393 = u32 13816530
            w405 = TRUE ("Visible")
            w407 = ""
            n253 = property on="ConfigName" class="Str"("Value"=w407) -> (error out=w403:errorcluster)  [unwired: 2 in, 1 out]
            n254 = property on="Text" class="Str"(error in=w403, "Value"=w407, "Visible"=w405) -> (error out=w404:errorcluster)  [unwired: 1 in, 1 out]
            n255 = property on="Components" class="MCListbox (strict)"("ItemNames"=string[][] [] ("Item Names"), "Value"=-1 ("Properties"), "TopLeft"=T16 {"Row"=0, "Column"=0} ("Top Left Visible Cell"), "ActiveCell"=T15 {"Row"=-2, "Column"=-2} ("Active Cell:Active Cell"), "CellBG"=u32 16777225, "ActiveCell"=T15 {"Row"=-1, "Column"=-2} ("Active Cell:Active Cell"), "CellBG"=w393, "ActiveCell"=T15 {"Row"=-2, "Column"=-1} ("Active Cell:Active Cell"), "CellBG"=w393, "CellFontColor"=u32 0) -> ()  [unwired: 2 in, 2 out]
            n256 = property on="Variable" class="Enum (strict)"(error in=w404, "Value"=DMCConfiguatorGui.VarGui."-" ("Variable"), "Visible"=w405) -> (error out=w402:errorcluster)  [unwired: 1 in, 1 out]
            n257 = property on="ConfigInUse" class="Ring (strict)"(error in=w402, "Strings []"=string[] [], "Value"=0) -> ()  [unwired: 1 in, 2 out]
          }
          frame #1 {
            n258 = call "Translator.TranslateThis.Exit.vi"("error in"=w410) -> ("error out"=w411:errorcluster)  [unwired: 10 in]
          }
        }
        n259 = property class="Pnl"(reference=w387, "DeferPanUpdts"=FALSE ("Defer Panel Updates")) -> (reference out=w389:refnum<vi>, error out=w390:errorcluster)  [unwired: 1 in]
        n260 = Close Reference(reference=w389, error in (no error)=w390) -> ()  [unwired: 1 out]
      }
      frame "--- DMC.Config.Gui ---" {
        # "--> Handle error here..."
        n261 = Unflatten From String(type=T18 {"ts"=timestamp(0 s since 1904-01-01), "src"=enum."All", "instance"=0, "action"="", "error"={"status"=FALSE, "code"=0, "source"=""}, "unconfirmed"=FALSE} ("ErrData"), binary string=w418, error in (no error)=w416) -> (value=w414:T18)  [unwired: 4 out]
        n262 = Unbundle By Name(w414) -> ("error"=w413:errorcluster)
        n263 = call <vilib>:"Clear Errors.vi"("error in (no error)"=w413) -> ("error out"=w417:errorcluster)  [unwired: 5 in, 1 out]
      }
      frame "open" {
        w422 = T14."Disabled and Grayed Out" ("Disabled")
        n264 = Unflatten From String(type=cluster{"Plate":T1, "OrderSets":T2} {"Plate"=enum."Wabco", "OrderSets"={"State"=enum."Init", "ImgPath"=path "", "WabcoPlate"="", "WabcoProduct"="", "ClientProduct"="", "ClientPlate"="", "TotalQuantity"=0, "OrderQuantity"=0, "Serial"=0, "Wabco"={"LaserJob"="", "AdditionalTxt"="", "FactoryCode"="", "RevID"=0, "ForkID"=0, "FailuresLimit"=0, "GlobalCnt"=0, "ScannerProgram"=0, "SerialFormat"=enum."", "CoordA"={"X"=0.0, "Y"=0.0, "Angle"=0.0}, "CoordB"={"X"=0.0, "Y"=0.0, "Angle"=0.0}, "DMCconfig"=0, "CVX_Program"=0}, "Client"={"LaserJob"="", "AdditionalTxt"="", "FactoryCode"="", "RevID"=0, "ForkID"=0, "FailuresLimit"=0, "GlobalCnt"=0, "ScannerProgram"=0, "SerialFormat"=enum."", "CoordA"={"X"=0.0, "Y"=0.0, "Angle"=0.0}, "CoordB"={"X"=0.0, "Y"=0.0, "Angle"=0.0}, "DMCconfig"=0, "CVX_Program"=0}}} ("output cluster"), binary string=w431, error in (no error)=w430) -> (value=w428:cluster{"Plate":T1, "OrderSets":T2}, error out=w423:errorcluster)  [unwired: 3 out]
        n265 = Unbundle(w428) -> ("Plate"=w427:T1, "OrderSets"=w426:T2)
        "OrderSets" <- w426
        "Plate" <- w427
        n266 = case shown="Default" w427 {
          tunnel: w426 -> [w433 w435]
          tunnel: [w432 w434] -> w425
          frame "Client" {
            n267 = Unbundle By Name(w433) -> ("Client"=w432:T4)
          }
          frame Default {
            n268 = Unbundle By Name(w435) -> ("Wabco"=w434:T4)
          }
        }
        n269 = property on="ConfigAdd" class="Bool"("DisabledEnum"=w422) -> ()  [unwired: 2 in, 2 out]
        n270 = property on="ConfigInUse" class="Ring (strict)"("DisabledEnum"=w422) -> ()  [unwired: 2 in, 2 out]
        n271 = Unbundle By Name(w425) -> ("DMCconfig"=w424:i32)
        "DMCconfig" <- w424
        n272 = property on="Hider" class="Bool (strict)"("Visible"=TRUE) -> ()  [unwired: 2 in, 2 out]
        n273 = property on="ConfigInUse" class="Ring (strict)"("Val(Sgnl)"=w424) -> ()  [unwired: 2 in, 2 out]
      }
      frame "update dmc" {
        n274 = Index Array(array=w460, index=w444) -> (element=w448:T7)
        n275 = Unbundle By Name(w448) -> ("Components"=w454:T8[])
        n276 = Equal To 0?(x=w444) -> (x = 0?=w443:bool)
        n277 = local read "OrderSets"() -> (w452:T2)
        n278 = local read "Plate"() -> (w453:T1)
        n279 = for {
          tunnel: w454 -> [w472] mode=indexing
          tunnel: w453 -> [w471]
          tunnel: w452 -> [w470]
          tunnel: [w469] -> w446 mode=indexing
          tunnel: w443 -> [w468]
          n280 = call "Sequence.Test.DMC.GetComponent.vi"("Default"=w468, "Component"=w472, "Plate"=w471, "OrderSets"=w470) -> ("size"=w469:i32)  [unwired: 5 in, 2 out]
        }
        n281 = call "Sequence.Test.CreateDMC.vi"("Default"=w443, "GUI? (F)"=TRUE, "DMCConfig"=w448, "Plate"=w453, "Variant"=w452) -> ("DMC"=w455:string)  [unwired: 5 in, 1 out]
        "DMC" <- w455
        n282 = call "Sequence.Test.DMC.GetDMCSize.vi"() -> ("max size"=w436:i32)  [unwired: 11 in]
        n283 = Format Into String(format string="DMC (#%d)" ("Caption.Text"), w436) -> (resulting string=w437:string)  [unwired: 2 in, 1 out]
        n284 = String Length(string=w455) -> (length=w459:i32)
        n285 = Index Array(array=w446, index=w447) -> (element=w445:i32)
        n286 = Array Subset(array=w446, length=w447) -> (w450:i32[])  [unwired: 1 in]
        n287 = property on="DMC" class="Str"("Caption.Text"=w437, "Text.Selection Start"=u32 0 ("Text.Selection:Start"), "Text.Selection End"=w459, "Text.FontColor"=u32 0) -> (error out=w449:errorcluster)  [unwired: 2 in, 1 out]
        n288 = Add Array Elements(numeric array=w450) -> (sum=w439:i32)
        n289 = Greater Or Equal To 0?(x=w447) -> (x >= 0?=w451:bool)
        n290 = Compound Arithmetic op=ADD(w439, w445) -> (w440:i32)
        n291 = Greater?(x=w440, y=w439) -> (0:w441:bool)
        n292 = Compound Arithmetic op=AND(w441, w451) -> (w442:bool)
        n293 = case shown="True" w442 {
          tunnel: w439 -> [_ w467]
          tunnel: w440 -> [_ w466]
          tunnel: w449 -> [w462 w465]
          tunnel: [w462 w463] -> _
          frame False {
          }
          frame True {
            n294 = property on="DMC" class="Str"(error in=w465, "Text.Selection Start"=w467, "Text.Selection End"=w466, "Text.FontColor"=u32 16711680) -> (error out=w463:errorcluster)  [unwired: 1 in, 1 out]
          }
        }
      }
      frame "load configurations" {
        n295 = for {
          tunnel: w482 -> [w486] mode=indexing
          tunnel: [w485] -> w483 mode=indexing
          n296 = Unbundle By Name(w486) -> ("Name"=w485:string)
        }
        n297 = property on="ConfigInUse" class="Ring (strict)"() -> ("Value"=w475:i32)  [unwired: 2 in, 2 out]
        n298 = Array Size(array=w483) -> (size(s)=w481:i32)
        n299 = Decrement(x=w481) -> (x-1=w479:i32)
        n300 = Less Or Equal To 0?(x=w479) -> (x <= 0?=w474:bool)
        n301 = In Range and Coerce(upper limit=w479, x=w475, lower limit=0) -> (coerced(x)=w478:i32)  [unwired: 1 out]
        n302 = Select(t=T14."Disabled and Grayed Out" ("Disabled"), s=w474, f=T14."Enabled" ("Disabled")) -> (s? t:f=w473:T14)
        n303 = property on="ConfigDelete" class="Bool"("DisabledEnum"=w473) -> ()  [unwired: 2 in, 2 out]
        n304 = property on="ConfigInUse" class="Ring (strict)"("Strings []"=w483, "Val(Sgnl)"=w478) -> ()  [unwired: 2 in, 2 out]
      }
      frame "accept" {
        n305 = call "ChangeOverGui-DMCAccept.vi"("error in"=w489, "Configuration"=w487) -> ("error out"=w488:errorcluster)  [unwired: 9 in]
      }
    }
    "ConfigData" <- w5
    n306 = call "citTemplate.sendAckNotifier.vi"("notification data"=w14, "notifierHandle in"=w15, "error in"=w12) -> ()  [unwired: 13 out]
    n307 = call "citTemplate.ErrorEventPass.vi"("error in"=w12, "action of error"=w9, "event in"=w13) -> ("error out"=w8:errorcluster)  [unwired: 2 in, 6 out]
  }
